vi "stage controller.vi"() -> ()   [LabVIEW 2016]
doc: "This VI allows manual control of the Mad City piezo stage. It also receives commands from the Command Stage Controller VI and moves the stage accordingly. Therefore, stage controller.vi must be RUNNING for the stage to respond to those commands."
uses:
  Move stage command.ctl
  new-h-nu-ixon/stage globals.vi
panel:
  out "Curr. Z":dbl(slide) scale=0.0..178.0
  out "Current (X,Y)":cluster{ext[], ext[]}(graph)
  out "At limit 3":bool
  out "At limit 2":bool
  out "At limit":bool
  in  "z-":bool
  in  "z step (um)":ext=0.1 format="%_5g"
  in  "z+":bool
  in  "x-":bool
  in  "x+":bool
  in  "y-":bool
  in  "x,y step (um)":ext=10.0 format="%_5g"
  in  "y+":bool
  out "Current Z (um)":ext=50.0 format="%_5g"
  out "Current Y (um)":ext=50.0 format="%_5g"
  out "Current X (um)":ext=50.0 format="%_5g"
  in  "Stop":bool
  in  "Reset stage to center\n(x, y, and z)":bool
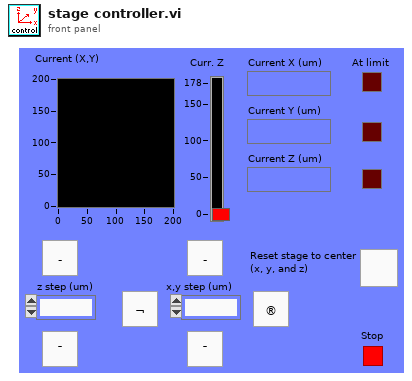
[diagram p1: front panel]
types:
  T1 = typedef "Move stage command.ctl" = cluster{"dx (um) (0 -> ignore)":ext, "dy (um) (0 -> ignore)":ext, "dz (um) (0 -> ignore)":ext, "Re-center x,y":bool, "Re-center z":bool, "x (um) (-1 -> ignore)":dbl, "y (um) (-1 -> ignore)":dbl, "z (um) (-1 -> ignore)":dbl}
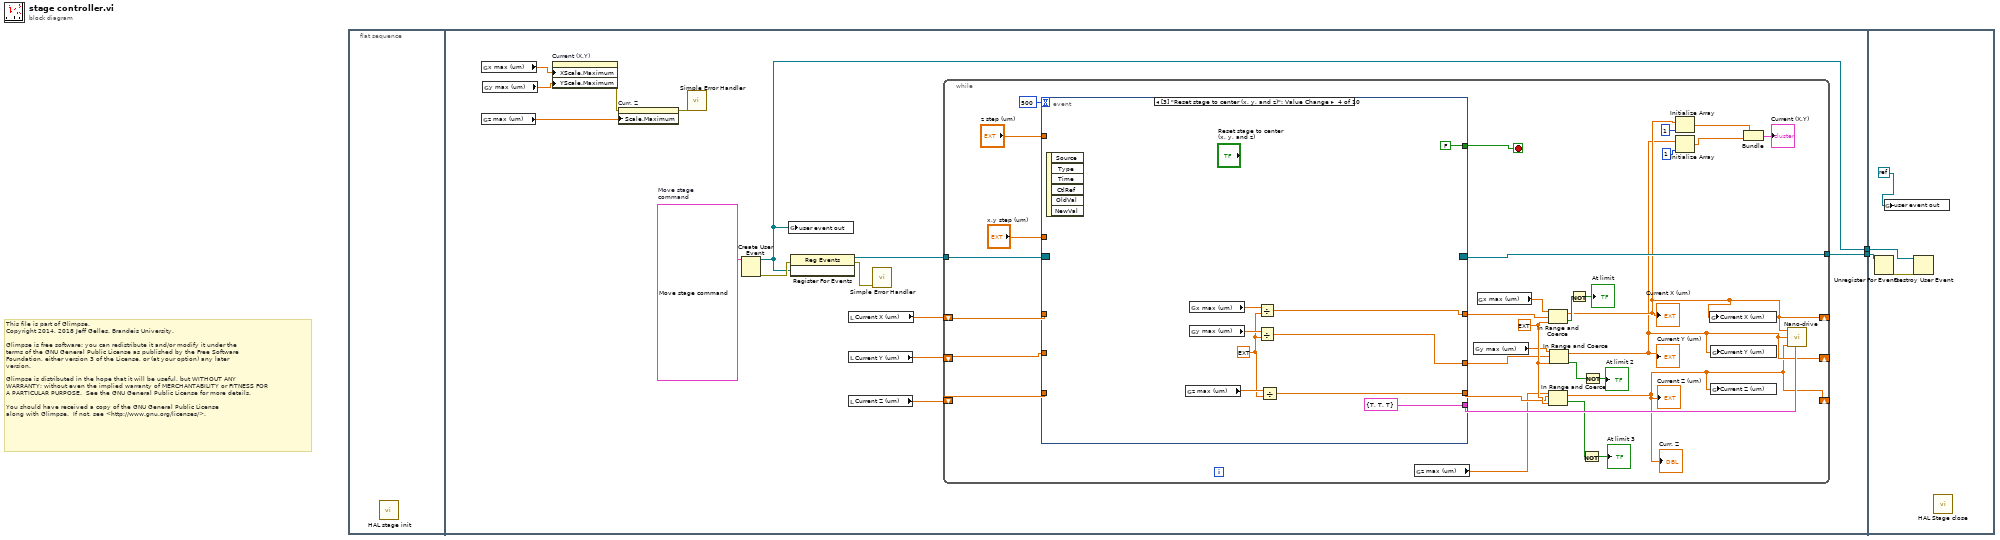
[diagram p0: block diagram]
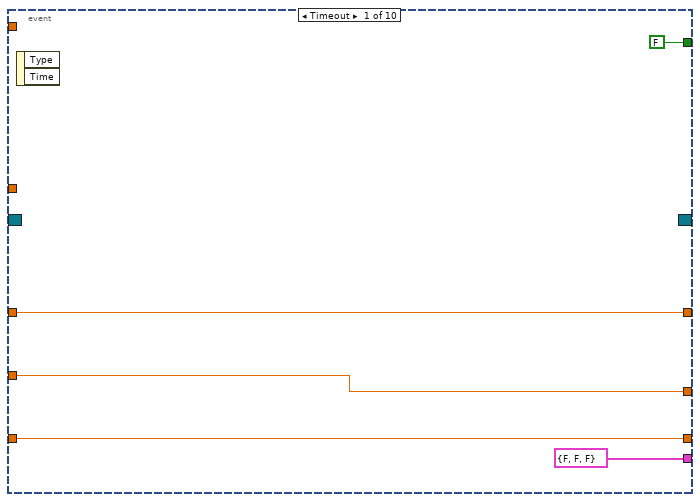
[diagram p2: hidden frame]
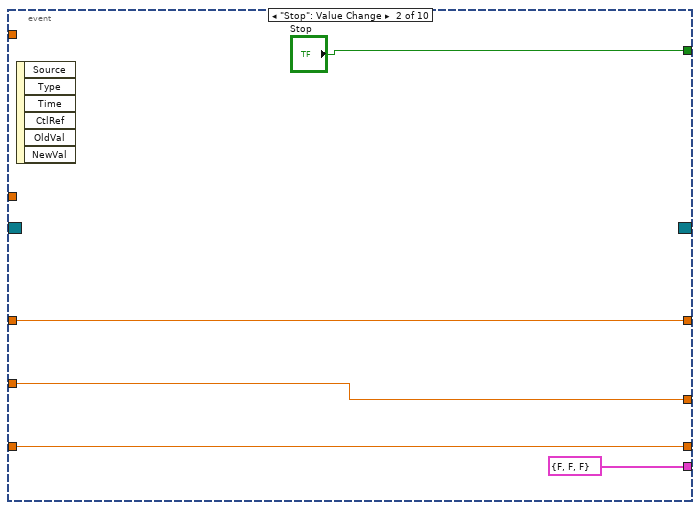
[diagram p3: hidden frame]
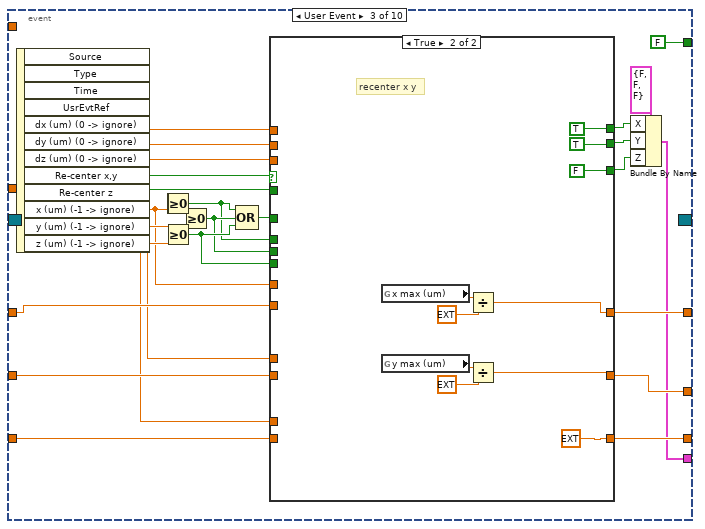
[diagram p4: hidden frame]
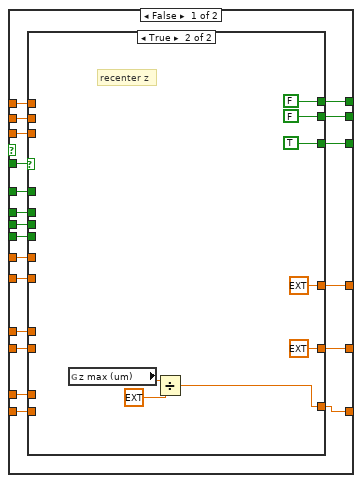
[diagram p5: hidden frame]
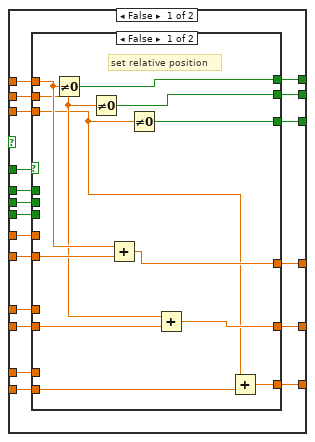
[diagram p6: hidden frame]
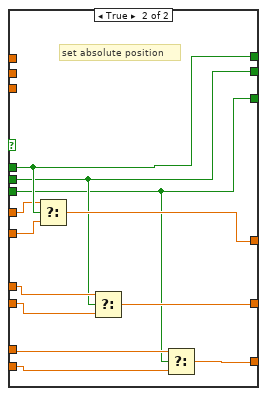
[diagram p7: hidden frame]
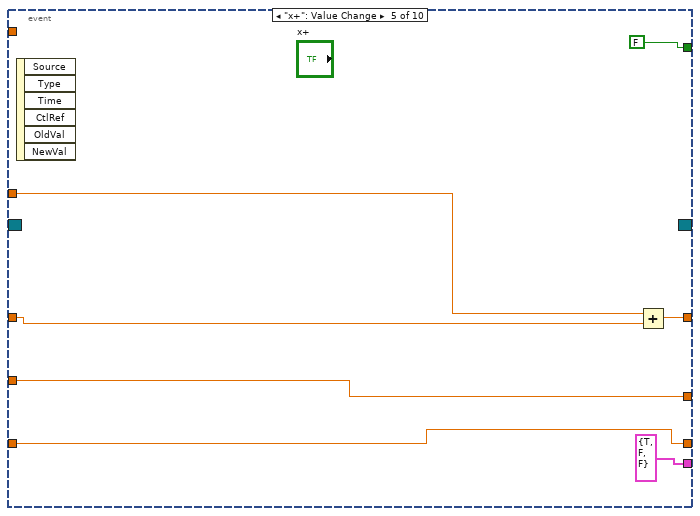
[diagram p8: hidden frame]
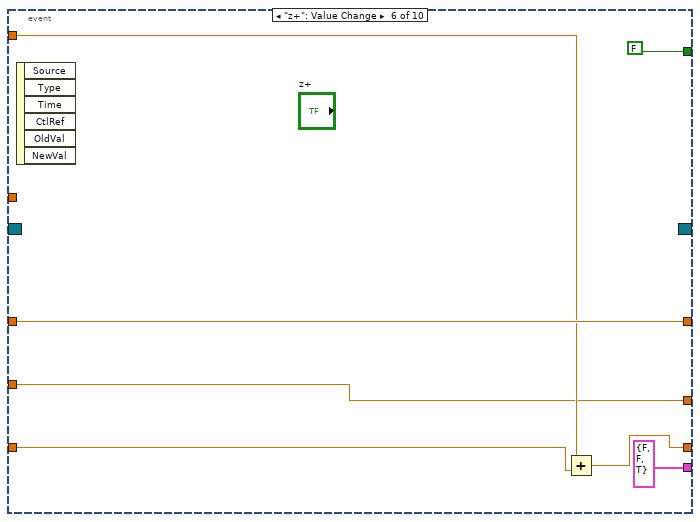
[diagram p9: hidden frame]
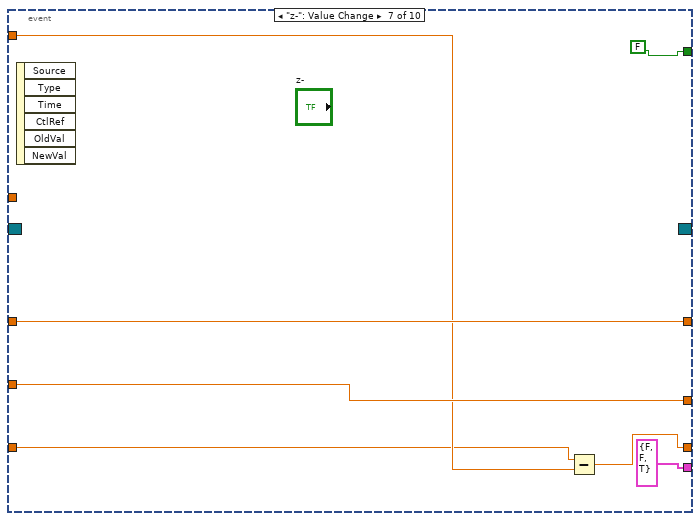
[diagram p10: hidden frame]
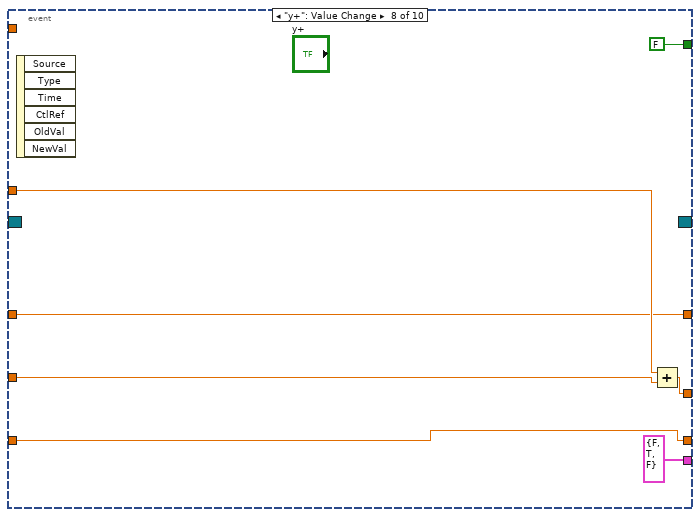
[diagram p11: hidden frame]
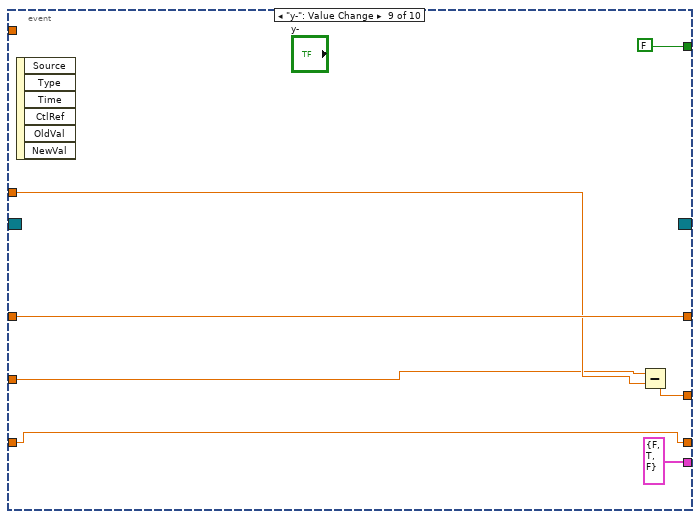
[diagram p12: hidden frame]
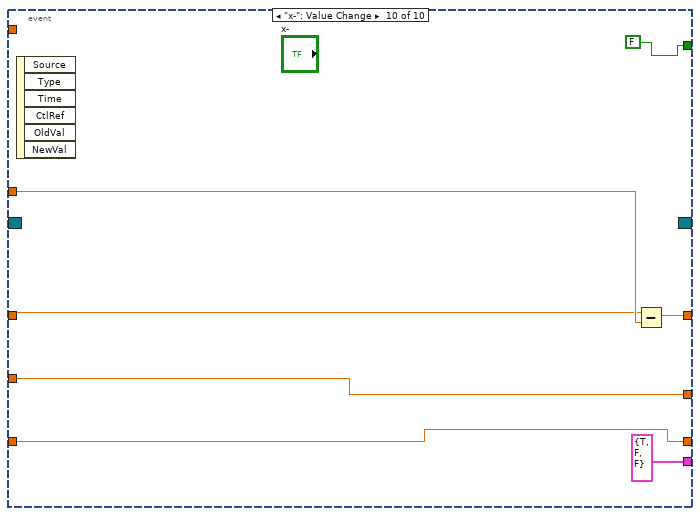
[diagram p13: hidden frame]
diagram:
  # "This file is part of Glimpse. \nCopyright 2014, 2018 Jeff Gelles, Brandeis University.    \n\nGlimpse is free software: you can redistribute it and/or modify it under the \nterms of the GNU General Public License as published by the Free Software \nFoundation, either version 3 of the License, or (at your option) any later \nversion.\n\nGlimpse is distributed in the hope that it will be useful, but WITHOUT ANY \nWARRANTY; without even the implied warranty of MERCHANTABILITY or FITNESS FOR \nA PARTICULAR PURPOSE.  See the GNU General Public License for more details.\n\nYou should have received a copy of the GNU General Public License\nalong with Glimpse.  If not, see <http://www.gnu.org/licenses/>."
  n1 = flat-sequence {
    tunnel: [w9] -> w2
    tunnel: [w8] -> w1
    tunnel: w2 -> [w217]
    tunnel: w1 -> [w214]
    frame #0 {
      n2 = call "HAL stage init.vi"() -> ()  [unwired: 1 in]
    }
    frame #1 {
      w13 = T1 {"dx (um) (0 -> ignore)"=0.0, "dy (um) (0 -> ignore)"=0.0, "dz (um) (0 -> ignore)"=0.0, "Re-center x,y"=FALSE, "Re-center z"=FALSE, "x (um) (-1 -> ignore)"=-1.0, "y (um) (-1 -> ignore)"=-1.0, "z (um) (-1 -> ignore)"=-1.0}  # Move stage command
      n3 = global read "stage globals.vi" "z max (um)"() -> (w6:ext)
      n4 = global read "stage globals.vi" "x max (um)"() -> (w7:ext)
      n5 = global read "stage globals.vi" "y max (um)"() -> (w3:ext)
      n6 = property on="Current (X,Y)" class="XYGraph (strict)"("XScale.Maximum"=w7, "YScale.Maximum"=w3) -> (error out=w5:errorcluster)  [unwired: 2 in, 1 out]
      n7 = property on="Curr. Z" class="Slide (strict)"(error in=w5, "Scale.Maximum"=w6) -> (error out=w4:errorcluster)  [unwired: 1 in, 1 out]
      n8 = call <vilib>:"Simple Error Handler.vi"("error in (no error)"=w4) -> ()  [unwired: 1 in, 8 out]
      n9 = Create User Event(user event datatype=w13) -> (user event=w8:refnum<user-event>, error out=w11:errorcluster)  [unwired: 1 in]
      n10 = global write "stage globals.vi" "user event out"(w8) -> ()
      n11 = register-events(error in=w11, w8) -> (reference out=w12:refnum<event-registration>, error out=w10:errorcluster)  [unwired: 1 in]
      n12 = local read "Current Y (um)"() -> (w15:ext)
      n13 = local read "Current Z (um)"() -> (w14:ext)
      n14 = local read "Current X (um)"() -> (w16:ext)
      n15 = call <vilib>:"Simple Error Handler.vi"("error in (no error)"=w10) -> ()  [unwired: 1 in, 8 out]
      n16 = while {
        shift-right: [w20] -> _
        shift-left: w16 -> [w34]
        shift-right: [w19] -> _
        shift-left: w15 -> [w33]
        shift-right: [w18] -> _
        shift-left: w14 -> [w32]
        tunnel: w12 -> [w45]
        tunnel: [w41] -> w9
        stop <- w47 stop-if-true
        w42 = ext 0.0 ("lower limit")
        n17 = event shown="[3] \"Reset stage to center (x, y, and z)\": Value Change" {
          selector: w45 -> [_ _ _ _ _ _ _ _ _ _]
          dyn-events: [_ _ _ _ _ _ _ _ _ _] -> w41
          timeout: 500 -> [_ _ _ _ _ _ _ _ _ _]
          tunnel: [FALSE ("Stop") "Stop" FALSE ("Stop") FALSE ("Stop") FALSE ("Stop") FALSE ("Stop") FALSE ("Stop") FALSE ("Stop") FALSE ("Stop") FALSE ("Stop")] -> w47
          tunnel: w34 -> [w51 w56 w81 _ w175 w184 w190 w194 w203 w210]
          tunnel: w33 -> [w50 w55 w80 _ w174 w179 w189 w196 w200 w209]
          tunnel: w32 -> [w49 w54 w79 _ w173 w181 w186 w198 w204 w208]
          tunnel: [w51 w56 w76 w163 w177 w184 w190 w194 w203 w212] -> w31
          tunnel: [w50 w55 w77 w168 w174 w179 w189 w197 w205 w209] -> w30
          tunnel: [w49 w54 w78 w167 w173 w183 w192 w198 w204 w208] -> w29
          tunnel: [cluster{"X":bool, "Y":bool, "Z":bool} {"X"=FALSE, "Y"=FALSE, "Z"=FALSE} ("Set this axis?") cluster{"X":bool, "Y":bool, "Z":bool} {"X"=FALSE, "Y"=FALSE, "Z"=FALSE} ("Set this axis?") w69 cluster{"X":bool, "Y":bool, "Z":bool} {"X"=TRUE, "Y"=TRUE, "Z"=TRUE} ("Set this axis?") cluster{"X":bool, "Y":bool, "Z":bool} {"X"=TRUE, "Y"=FALSE, "Z"=FALSE} ("Set this axis?") cluster{"X":bool, "Y":bool, "Z":bool} {"X"=FALSE, "Y"=FALSE, "Z"=TRUE} ("Set this axis?") cluster{"X":bool, "Y":bool, "Z":bool} {"X"=FALSE, "Y"=FALSE, "Z"=TRUE} ("Set this axis?") cluster{"X":bool, "Y":bool, "Z":bool} {"X"=FALSE, "Y"=TRUE, "Z"=FALSE} ("Set this axis?") cluster{"X":bool, "Y":bool, "Z":bool} {"X"=FALSE, "Y"=TRUE, "Z"=FALSE} ("Set this axis?") cluster{"X":bool, "Y":bool, "Z":bool} {"X"=TRUE, "Y"=FALSE, "Z"=FALSE} ("Set this axis?")] -> w46
          tunnel: "x,y step (um)" -> [_ _ _ _ w176 _ _ w195 w201 w211]
          tunnel: "z step (um)" -> [_ _ _ _ _ w180 w187 _ _ _]
          event Timeout {
            n18 = event-data() -> ()  [unwired: 3 out]
          }
          event "Stop": Value Change {
            n19 = event-data() -> ()  [unwired: 7 out]
          }
          event User Event {
            n20 = event-data() -> ("dx (um) (0 -> ignore)"=w74:ext, "dy (um) (0 -> ignore)"=w73:ext, "dz (um) (0 -> ignore)"=w72:ext, "Re-center x,y"=w71:bool, "Re-center z"=w65:bool, "x (um) (-1 -> ignore)"=w61:dbl, "y (um) (-1 -> ignore)"=w62:dbl, "z (um) (-1 -> ignore)"=w63:dbl)  [unwired: 5 out]
            n21 = Greater Or Equal To 0?(x=w61) -> (x >= 0?=w58:bool)
            n22 = Greater Or Equal To 0?(x=w61) -> ()  [unwired: 1 out]
            n23 = Greater Or Equal To 0?(x=w63) -> (x >= 0?=w60:bool)
            n24 = Greater Or Equal To 0?(x=w62) -> (x >= 0?=w59:bool)
            n25 = Compound Arithmetic op=OR(w58, w59, w60) -> (w64:bool)
            n26 = case shown="True" w71 {
              tunnel: w81 -> [w101 _]
              tunnel: w80 -> [w100 _]
              tunnel: w79 -> [w99 _]
              tunnel: [w98 ext 0.0] -> w78
              tunnel: [w97 w153] -> w77
              tunnel: [w96 w156] -> w76
              tunnel: w74 -> [w95 _]
              tunnel: w73 -> [w94 _]
              tunnel: w72 -> [w93 _]
              tunnel: [w92 FALSE] -> w68
              tunnel: [w91 TRUE] -> w67
              tunnel: [w90 TRUE] -> w66
              tunnel: w65 -> [w89 _]
              tunnel: w64 -> [w88 _]
              tunnel: w63 -> [w87 _]
              tunnel: w62 -> [w86 _]
              tunnel: w61 -> [w85 _]
              tunnel: w60 -> [w84 _]
              tunnel: w59 -> [w83 _]
              tunnel: w58 -> [w82 _]
              frame False {
                n27 = case shown="True" w89 {
                  tunnel: w101 -> [w120 _]
                  tunnel: w100 -> [w119 _]
                  tunnel: w99 -> [w118 _]
                  tunnel: [w117 w150] -> w98
                  tunnel: [w116 ext 0.0] -> w97
                  tunnel: [w115 ext 0.0] -> w96
                  tunnel: w95 -> [w114 _]
                  tunnel: w94 -> [w113 _]
                  tunnel: w93 -> [w112 _]
                  tunnel: [w111 TRUE] -> w92
                  tunnel: [w110 FALSE] -> w91
                  tunnel: [w109 FALSE] -> w90
                  tunnel: w88 -> [w108 _]
                  tunnel: w87 -> [w107 _]
                  tunnel: w86 -> [w106 _]
                  tunnel: w85 -> [w105 _]
                  tunnel: w84 -> [w104 _]
                  tunnel: w83 -> [w103 _]
                  tunnel: w82 -> [w102 _]
                  frame False {
                    n28 = case shown="False" w108 {
                      tunnel: w120 -> [w132 w140]
                      tunnel: w119 -> [w131 w137]
                      tunnel: w118 -> [w130 w134]
                      tunnel: [w129 w136] -> w117
                      tunnel: [w128 w139] -> w116
                      tunnel: [w127 w143] -> w115
                      tunnel: w114 -> [w126 _]
                      tunnel: w113 -> [w125 _]
                      tunnel: w112 -> [w124 _]
                      tunnel: [w123 w133] -> w111
                      tunnel: [w122 w138] -> w110
                      tunnel: [w121 w142] -> w109
                      tunnel: w107 -> [_ w135]
                      tunnel: w106 -> [_ w144]
                      tunnel: w105 -> [_ w141]
                      tunnel: w104 -> [_ w133]
                      tunnel: w103 -> [_ w138]
                      tunnel: w102 -> [_ w142]
                      frame False {
                        # "set relative position"
                        n29 = Not Equal To 0?(x=w126) -> (x != 0?=w121:bool)
                        n30 = Not Equal To 0?(x=w125) -> (x != 0?=w122:bool)
                        n31 = Add(x=w126, y=w132) -> (x+y=w127:ext)
                        n32 = Not Equal To 0?(x=w124) -> (x != 0?=w123:bool)
                        n33 = Add(x=w125, y=w131) -> (x+y=w128:ext)
                        n34 = Add(x=w124, y=w130) -> (x+y=w129:ext)
                      }
                      frame True {
                        # "set absolute position"
                        n35 = Select(t=w141, s=w142, f=w140) -> (s? t:f=w143:ext)
                        n36 = Select(t=w144, s=w138, f=w137) -> (s? t:f=w139:ext)
                        n37 = Select(t=w135, s=w133, f=w134) -> (s? t:f=w136:ext)
                      }
                    }
                  }
                  frame True {
                    # "recenter z"
                    n38 = global read "stage globals.vi" "z max (um)"() -> (w152:ext)
                    n39 = Divide(x=w152, y=ext 2.0) -> (x/y=w150:ext)
                  }
                }
              }
              frame True {
                # "recenter x y"
                n40 = global read "stage globals.vi" "x max (um)"() -> (w161:ext)
                n41 = global read "stage globals.vi" "y max (um)"() -> (w155:ext)
                n42 = Divide(x=w161, y=ext 2.0) -> (x/y=w156:ext)
                n43 = Divide(x=w155, y=ext 2.0) -> (x/y=w153:ext)
              }
            }
            n44 = Bundle By Name(cluster=cluster{"X":bool, "Y":bool, "Z":bool} {"X"=FALSE, "Y"=FALSE, "Z"=FALSE} ("Set this axis?"), "X"=w66, "Y"=w67, "Z"=w68) -> (w69:cluster{"X":bool, "Y":bool, "Z":bool})
          }
          event "Reset stage to center\n(x, y, and z)": Value Change {
            w164 = ext 2.0 ("y")
            n45 = event-data() -> ()  [unwired: 7 out]
            n46 = global read "stage globals.vi" "z max (um)"() -> (w169:ext)
            n47 = global read "stage globals.vi" "x max (um)"() -> (w165:ext)
            n48 = global read "stage globals.vi" "y max (um)"() -> (w166:ext)
            n49 = Divide(x=w165, y=w164) -> (x/y=w163:ext)
            n50 = Divide(x=w166, y=w164) -> (x/y=w168:ext)
            n51 = Divide(x=w169, y=w164) -> (x/y=w167:ext)
          }
          event "x+": Value Change {
            n52 = event-data() -> ()  [unwired: 7 out]
            n53 = Add(x=w176, y=w175) -> (x+y=w177:ext)
          }
          event "z+": Value Change {
            n54 = event-data() -> ()  [unwired: 7 out]
            n55 = Add(x=w180, y=w181) -> (x+y=w183:ext)
          }
          event "z-": Value Change {
            n56 = event-data() -> ()  [unwired: 7 out]
            n57 = Subtract(x=w186, y=w187) -> (x-y=w192:ext)
          }
          event "y+": Value Change {
            n58 = event-data() -> ()  [unwired: 7 out]
            n59 = Add(x=w195, y=w196) -> (x+y=w197:ext)
          }
          event "y-": Value Change {
            n60 = event-data() -> ()  [unwired: 7 out]
            n61 = Subtract(x=w200, y=w201) -> (x-y=w205:ext)
          }
          event "x-": Value Change {
            n62 = event-data() -> ()  [unwired: 7 out]
            n63 = Subtract(x=w210, y=w211) -> (x-y=w212:ext)
          }
        }
        n64 = global read "stage globals.vi" "z max (um)"() -> (w23:ext)
        n65 = global read "stage globals.vi" "y max (um)"() -> (w17:ext)
        n66 = global read "stage globals.vi" "x max (um)"() -> (w22:ext)
        n67 = In Range and Coerce(upper limit=w22, x=w31, lower limit=w42) -> (coerced(x)=w20:ext, In Range?=w39:bool)
        "Current X (um)" <- w20
        n68 = In Range and Coerce(upper limit=w23, x=w29, lower limit=w42) -> (coerced(x)=w18:ext, In Range?=w35:bool)
        "Current Z (um)" <- w18
        "Curr. Z" <- w18
        n69 = In Range and Coerce(upper limit=w17, x=w30, lower limit=w42) -> (coerced(x)=w19:ext, In Range?=w37:bool)
        "Current Y (um)" <- w19
        n70 = Not(x=w39) -> (.not. x?=→"At limit":bool)
        n71 = Not(x=w35) -> (.not. x?=→"At limit 3":bool)
        n72 = Not(x=w37) -> (.not. x?=→"At limit 2":bool)
        n73 = Initialize Array(w20, 1 ("dimension size")) -> (w26:ext[])
        n74 = Initialize Array(w19, 1 ("dimension size")) -> (w27:ext[])
        n75 = global write "stage globals.vi" "Current X (um)"(w20) -> ()
        n76 = global write "stage globals.vi" "Current Y (um)"(w19) -> ()
        n77 = global write "stage globals.vi" "Current Z (um)"(w18) -> ()
        n78 = Bundle(w26, w27) -> (→"Current (X,Y)":cluster{ext[], ext[]})  [unwired: 1 out]
        n79 = call "Nano-drive.vi"("X (um)"=w20, "Y (um)"=w19, "Z (um)"=w18, "Set this axis?"=w46) -> ()  [unwired: 5 out]
      }
    }
    frame #2 {
      n80 = Unregister For Events(event registration refnum=w217) -> (error out=w216:errorcluster)  [unwired: 1 in]
      n81 = global write "stage globals.vi" "user event out"(refnum<k0> refnum) -> ()
      n82 = Destroy User Event(user event=w214, error in=w216) -> ()  [unwired: 1 out]
      n83 = call "HAL Stage close.vi"() -> ()  [unwired: 12 in]
    }
  }
